vi "Intan_TeensyRestart.vi"(8 "error in":errorcluster, 10 "milliseconds to wait":u32=1000, 11 "VISA resource name":refnum<visa-resource-name>="COM1") -> (0 "error out":errorcluster, 1 "Reboot cmd response":string, 3 "VISA resource name out":refnum<visa-resource-name>)   [LabVIEW 2011]
doc: "Reboots Teensy, tests for USB link by attempting to write VISA resource.\nIf error is thrown, we need to reconnect. In this case, we close the current visa session,\nclear errors, then reinitiaize the serial port with the same VISA resource name"
panel:
  in  "event char (verify)":string="v"
  in  "restart event char  (Teensyduino)":string="p"
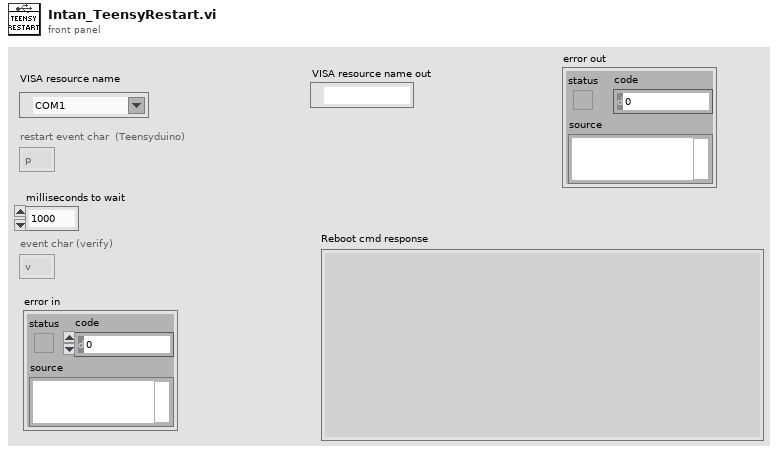
[diagram p1: front panel]
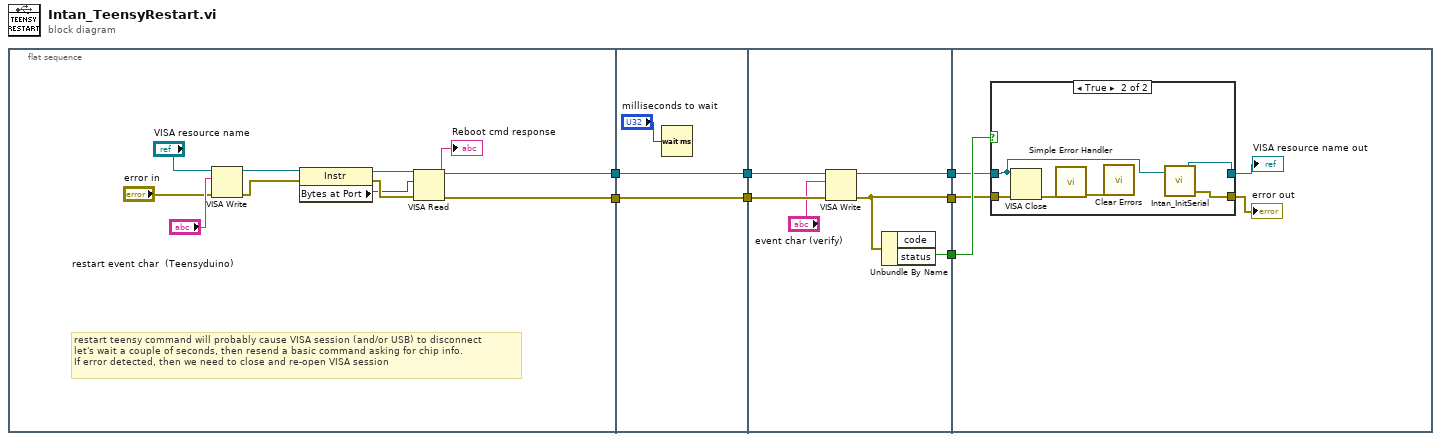
[diagram p0: block diagram]
diagram:
  n1 = flat-sequence {
    tunnel: [w9] -> w6
    tunnel: [w8] -> w4
    tunnel: [w20] -> w7
    tunnel: w6 -> [w20]
    tunnel: [w19] -> w5
    tunnel: w4 -> [w19]
    tunnel: w7 -> [w27]
    tunnel: w5 -> [w26]
    tunnel: [w24] -> w3
    tunnel: [w23] -> w2
    tunnel: [w22] -> w1
    tunnel: w3 -> [w32]
    tunnel: w2 -> [w31]
    tunnel: w1 -> [w30]
    frame #0 {
      # "restart teensy command will probably cause VISA session (and/or USB) to disconnect\nlet's wait a couple of seconds, then resend a basic command asking for chip info.\nIf error detected, then we need to close and re-open VISA session"
      n2 = VISA Write(VISA resource name="VISA resource name", write buffer="restart event char  (Teensyduino)", error in (no error)="error in") -> (VISA resource name out=w12:refnum<visa-resource-name>, error out=w11:errorcluster)  [unwired: 1 out]
      n3 = property class="Instr"(reference=w12, error in=w11) -> (reference out=w16:refnum<visa-resource-name>, error out=w15:errorcluster, "Bytes at Port"=w14:u32)
      n4 = VISA Read(VISA resource name=w16, byte count=w14, error in (no error)=w15) -> (VISA resource name out=w9:refnum<visa-resource-name>, read buffer=→"Reboot cmd response":string, error out=w8:errorcluster)  [unwired: 1 out]
    }
    frame #1 {
      n5 = Wait (ms)(milliseconds to wait="milliseconds to wait") -> ()  [unwired: 1 out]
    }
    frame #2 {
      n6 = VISA Write(VISA resource name=w27, write buffer="event char (verify)", error in (no error)=w26) -> (VISA resource name out=w23:refnum<visa-resource-name>, error out=w22:errorcluster)  [unwired: 1 out]
      n7 = Unbundle By Name(w22) -> ("status"=w24:bool)  [unwired: 1 out]
    }
    frame #3 {
      n8 = case shown="True" w32 {
        tunnel: w31 -> [w33 w37]
        tunnel: w30 -> [w34 w40]
        tunnel: [w33 w36] -> w29
        tunnel: [w34 w35] -> w28
        frame False {
        }
        frame True {
          n9 = VISA Close(VISA resource name=w37, error in (no error)=w40) -> (error out=w39:errorcluster)
          n10 = call <vilib>:"Simple Error Handler.vi"("error in (no error)"=w39) -> ("error out"=w38:errorcluster)  [unwired: 4 in, 4 out]
          n11 = call <vilib>:"Clear Errors.vi"("error in (no error)"=w38) -> ()  [unwired: 6 in, 1 out]
          n12 = call "Intan_InitSerial.vi"("VISA resource name"=w37) -> ("error out"=w35:errorcluster, "VISA resource name out"=w36:refnum<visa-resource-name>)  [unwired: 2 in, 1 out]
        }
      }
      "VISA resource name out" <- w29
      "error out" <- w28
    }
  }
